vi "cameraV1 teardown.vi"(8 "error in":errorcluster, 11 "Module ID":i32) -> (0 "error out":errorcluster)   [LabVIEW 2024]
doc: "_____\nCreated using DQMH Framework: Event Scripter 7.1.0.1503."
uses:
  Libraries/cameraV1/cameraV1.lvlib
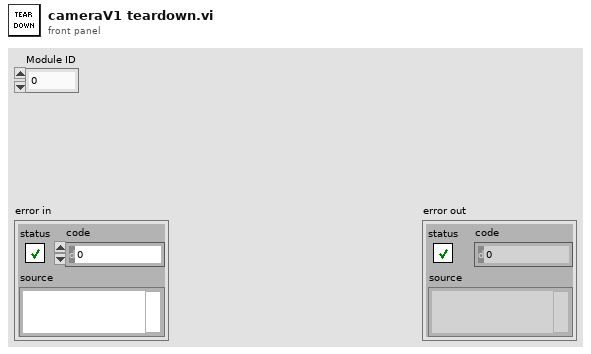
[diagram p1: front panel]
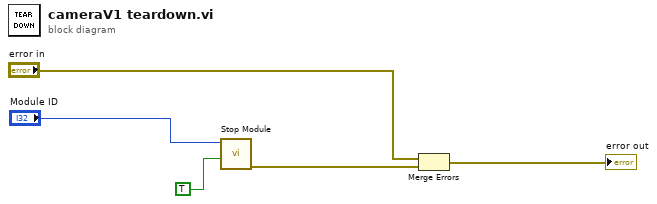
[diagram p0: block diagram]
diagram:
  n1 = call "Stop Module.vi"("Wait for Module to stop? (F)"=TRUE, "Module ID"="Module ID") -> ("error out"=w5:errorcluster)  [unwired: 9 in]
  n2 = Merge Errors("error in", w5) -> (→"error out":errorcluster)
